vi "Test TDS1002 Oscilloscope API.vi"() -> ()   [LabVIEW 2020]
doc: "TDS1002 Oscilloscope API Tester."
uses:
  Support/Channel configuration--cluster.ctl
  Trigger config--cluster.ctl
  <vilib>/Utility/error.llb/DialogType.ctl
  TDS1002 Oscilloscope.lvlib
panel:
  in  "Timebase":dbl=0.0005
  in  "Configure timebase":bool
  out "Measurements":dbl(graph)
  in  "Measurement Type":i32(ring) items=["Frequency", "Mean", "Period", "Pulse Duty", "Peak to Peak", "Cycle RMS", "Minimum", "Maximum", "Rise Time", "Fall Time", "Positive Width", "Negative Width", "Amplitude", "Cycle Mean", "High", "Low", "Negative Duty", "Positive Overshoot", "Negative Overshoot", "Cursor Mean", "Burst Width", "Positive Pulse Count", "Negative Pulse Count", "Rising Edge Count", "Falling Edge Count", "Area", "Cycle Area", "RMS", "Cursor RMS"]
  in  "Channel":i32(ring)=1 items=["Channel 1"=1, "Channel 2"=2, "Channel 3"=3, "Channel 4"=4]
  in  "Get measurement":bool
  out "Data from display":waveform(dbl)(graph)
  in  "Stop continuous acquisition":bool
  in  "Timeout":i32
  in  "Start continuous acquistion":bool
  in  "Send software trigger":bool
  in  "Trigger config":T1 {"Trigger Coupling" items=["AC", "DC", "HF Reject", "LF Reject", "Noise Reject"]; "Trigger Slope" items=["Rising", "Falling"]; "Trigger Mode" items=["Auto", "Normal"]; "Trigger Source" items=["Channel 1", "Channel 2", "Channel 3", "Channel 4", "External Input", "Attenuated External Input"]}
  in  "Configure trigger":bool
  in  "Config parameters":T2={"Acquisition Type"=0, "Averaged Waveforms"=4, "Channel"=0, "Probe Attenuation"=10, "Timebase"=0.0005} {"Probe Attenuation" items=["1"=1, "10"=10, "20"=20, "50"=50, "100"=100, "500"=500, "1000"=1000]; "Channel" items=["Channel 1", "Channel 2", "Channel 3", "Channel 4", "Math", "Reference A", "Reference B", "Reference C", "Reference D"]; "Averaged Waveforms" items=["4"=4, "16"=16, "64"=64, "128"=128]; "Acquisition Type" items=["Sample", "Average", "Peak Detect"]}
  in  "Type":enum16{"On demand", "Continous"}(ring)
  in  "Configure":bool
  in  "Disconnect":bool
  in  "VISA resource name":refnum<visa-resource-name>
  in  "Connect":bool
  in  "Remove Panel from Subpanel":bool
  in  "Draw Panel into Subpanel":bool
  in  "Show Diagram on Init":bool
  in  "Run as Singleton?":bool
  in  "Show Block Diagram":bool
  in  "Refresh Modules":bool
  out "Active Modules":string[](array[string])
  in  "Stop Module":bool
  in  "Select Module":i32(ring)=-1 caption="Select Module\nTo send Request to" items=["All"=-1]
  in  "Run New Module":bool
  in  "Hide Module Panel":bool
  in  "Show Module Panel":bool
  out "Status":string
  # "This VI tests the API for the Module."
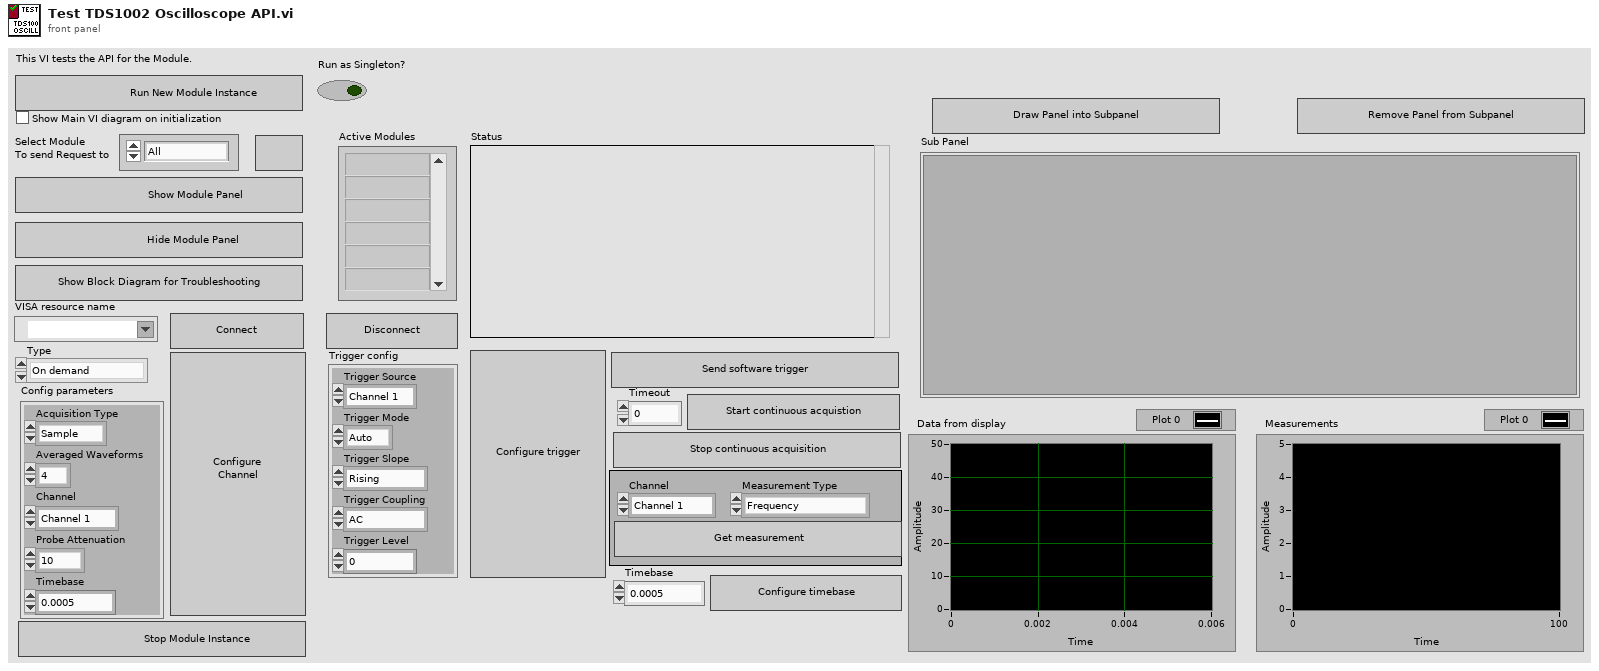
[diagram p1: front panel]
types:
  T1 = typedef "TDS1002 Oscilloscope.lvlib/Trigger config--cluster.ctl" = cluster{"Trigger Source":i32, "Trigger Mode":i32, "Trigger Slope":i32, "Trigger Coupling":i32, "Trigger Level":dbl}
  T2 = typedef "TDS1002 Oscilloscope.lvlib/Channel configuration--cluster.ctl" = cluster{"Acquisition Type":i32, "Averaged Waveforms":i32, "Channel":i32, "Probe Attenuation":i32, "Timebase":dbl}
  T3 = typedef "TDS1002 Oscilloscope.lvlib/Broadcast Events--cluster.ctl" = cluster{"Module Did Init":refnum<user-event>, "Status Updated":refnum<user-event>, "Error Reported":refnum<user-event>, "Module Did Stop":refnum<user-event>, "Update Module Execution Status":refnum<user-event>, "Helper Loop Status Updated":refnum<user-event>, "Device connected":refnum<user-event>, "Device disconnected":refnum<user-event>, "Data acquired":refnum<user-event>, "Configuration applied":refnum<user-event>}
  T4 = typedef "DialogType.ctl" = u16
  T5 = typedef "TDS1002 Oscilloscope.lvlib/Helper Loop Status--enum.ctl" = enum16{"Awake", "Asleep"}
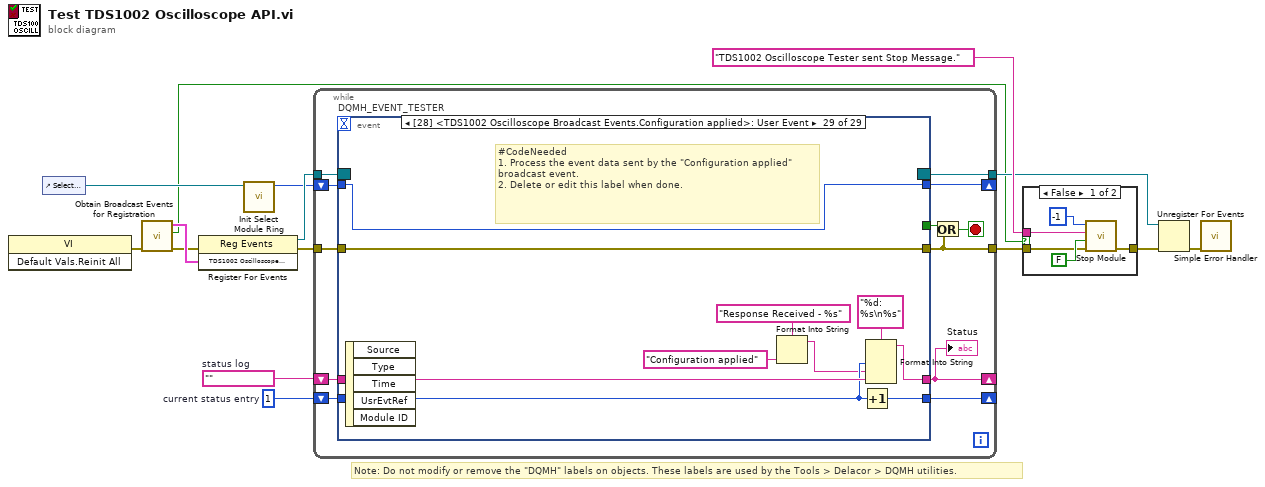
[diagram p0: block diagram]
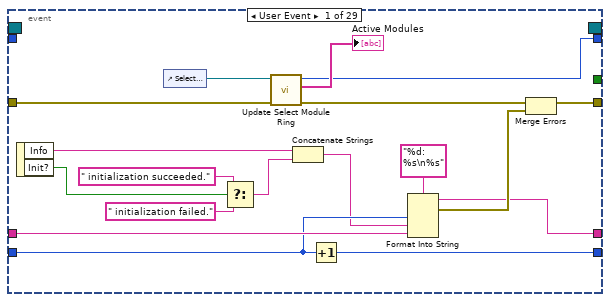
[diagram p3: hidden frame]
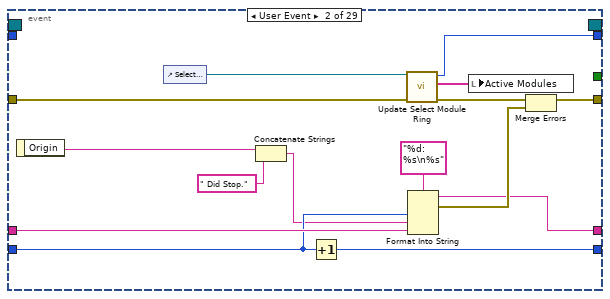
[diagram p4: hidden frame]
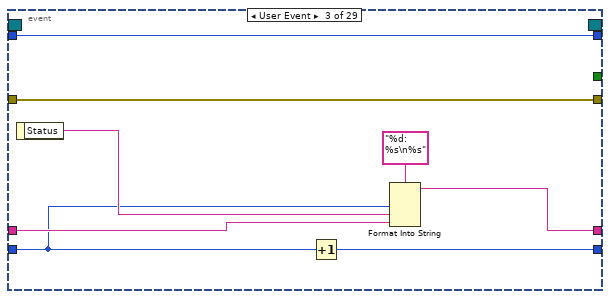
[diagram p5: hidden frame]
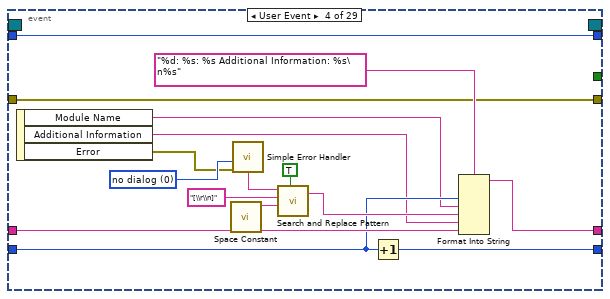
[diagram p6: hidden frame]
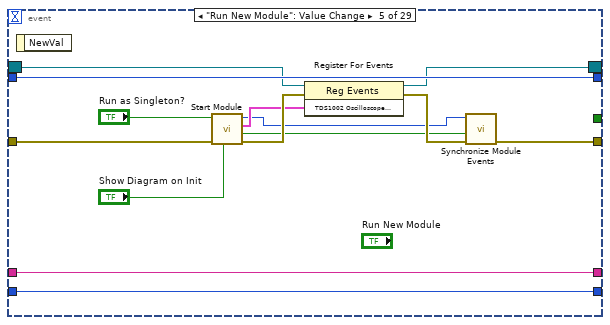
[diagram p7: hidden frame]
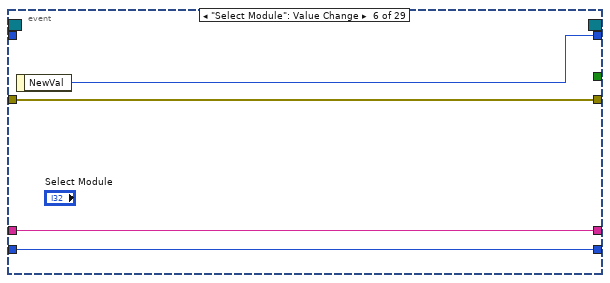
[diagram p8: hidden frame]
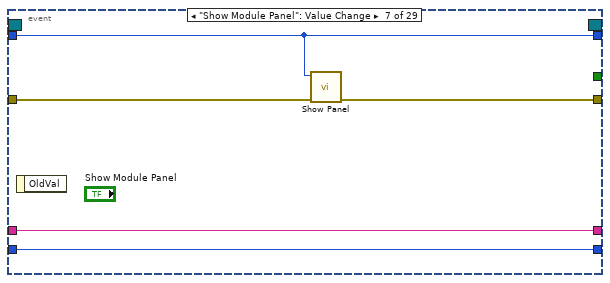
[diagram p9: hidden frame]
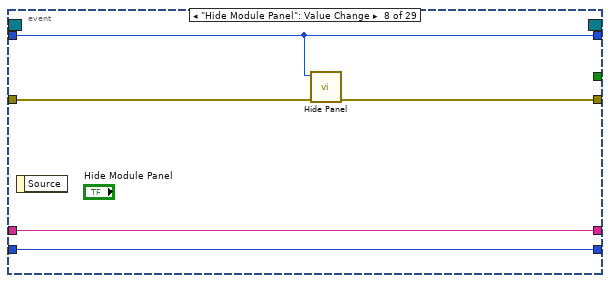
[diagram p10: hidden frame]
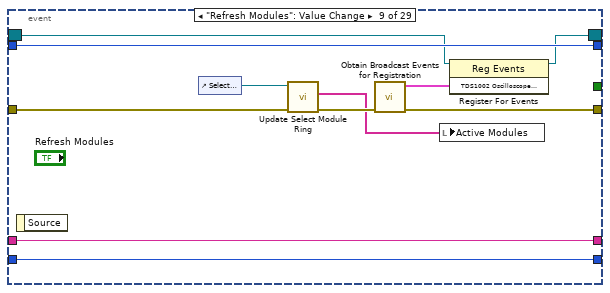
[diagram p11: hidden frame]
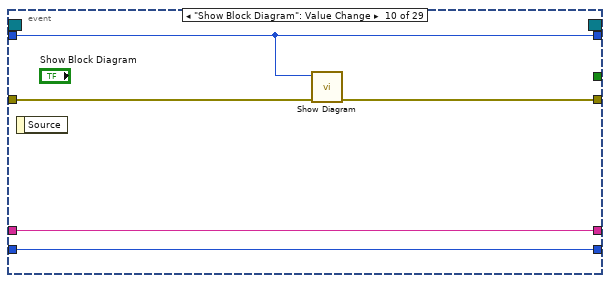
[diagram p12: hidden frame]
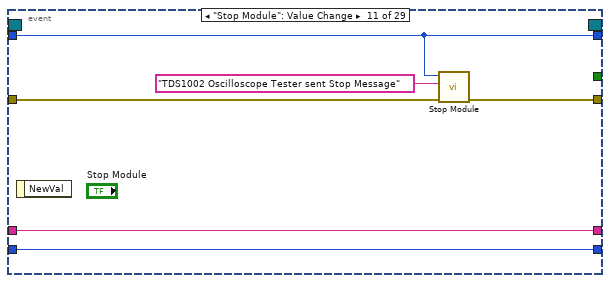
[diagram p13: hidden frame]
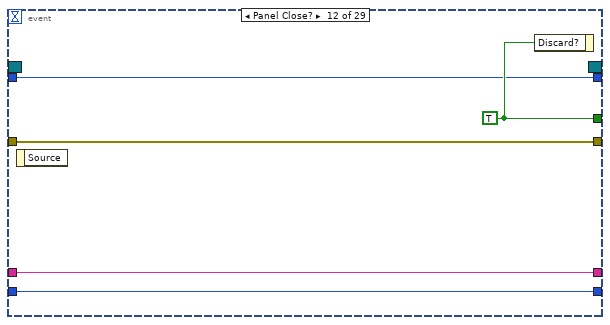
[diagram p14: hidden frame]
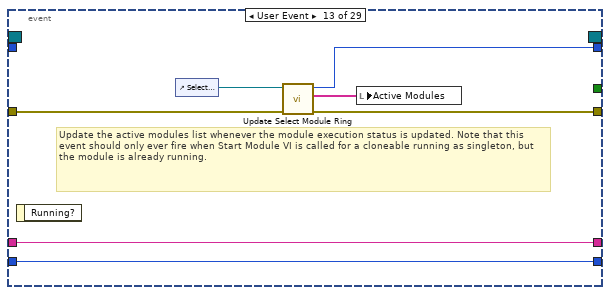
[diagram p15: hidden frame]
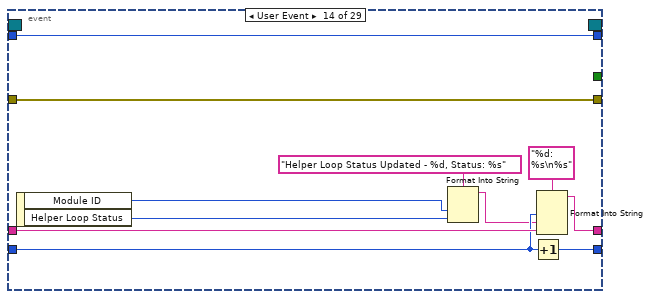
[diagram p16: hidden frame]
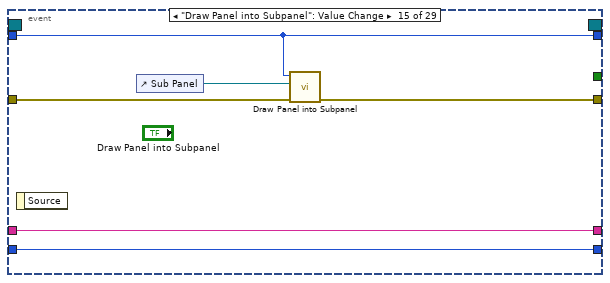
[diagram p17: hidden frame]
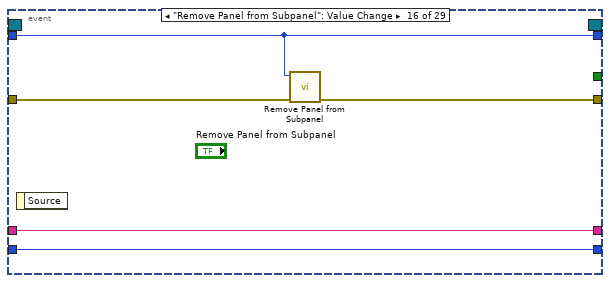
[diagram p18: hidden frame]
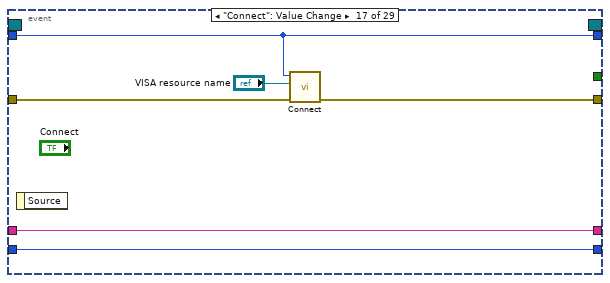
[diagram p19: hidden frame]
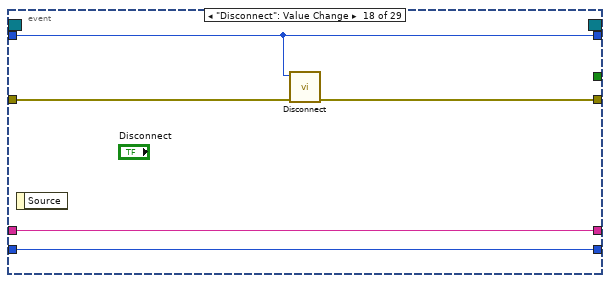
[diagram p20: hidden frame]
diagram:
  w12 = 1  # current status entry
  w13 = ""  # status log
  # "Note: Do not modify or remove the \"DQMH\" labels on objects. These labels are used by the Tools > Delacor > DQMH utilities."
  n1 = invoke class="VI" method="Default Vals.Reinit All"() -> (error out=w5:errorcluster)  [unwired: 3 in, 2 out]
  n2 = control-ref of="Select Module"() -> (w10:refnum<vi>)
  n3 = call "Obtain Broadcast Events for Registration.vi"("error in"=w5) -> ("error out"=w4:errorcluster, "Already running?"=w3:bool, "TDS1002 Oscilloscope Broadcast Events"=w9:T3)  [unwired: 8 in]
  n4 = register-events(error in=w4, w9) -> (reference out=w15:refnum<event-registration>, error out=w8:errorcluster)  [unwired: 1 in]
  n5 = call "Init Select Module Ring.vi"("Select Module Ring Ref"=w10) -> ("Value for All Modules"=w11:i32)  [unwired: 8 in, 2 out]
  n6 = while {
    tunnel: w15 -> [w27]
    tunnel: [w16] -> w2
    tunnel: w8 -> [w25]
    shift-right: [w21] -> _
    shift-left: w13 -> [w23]
    shift-right: [w22] -> _
    shift-left: w12 -> [w24]
    shift-right: [w18] -> _
    shift-left: w11 -> [w19]
    tunnel: [w17] -> w6
    stop <- w20 stop-if-true
    n7 = event "DQMH_EVENT_TESTER" shown="[28] <TDS1002 Oscilloscope Broadcast Events.Configuration applied>: User Event" {
      selector: w27 -> [_ _ _ _ w92 _ _ _ w118 _ _ _ _ _ _ _ _ _ _ _ _ _ _ _ _ _ _ _ _]
      dyn-events: [_ _ _ _ w91 _ _ _ w117 _ _ _ _ _ _ _ _ _ _ _ _ _ _ _ _ _ _ _ _] -> w17
      timeout: _ -> [_ _ _ _ _ _ _ _ _ _ _ _ _ _ _ _ _ _ _ _ _ _ _ _ _ _ _ _ _]
      tunnel: [_ _ _ _ _ _ _ _ _ _ _ w139 _ _ _ _ _ _ _ _ _ _ _ _ _ _ _ _ _] -> w26
      tunnel: [w35 w52 w68 w72 w90 w102 w106 w111 w114 w125 w130 w138 w142 w157 w160 w165 w171 w176 w189 w199 w203 w209 w214 w228 w231 w236 w244 w250 w263] -> w16
      tunnel: w25 -> [w37 w54 w68 w72 w93 w102 w107 w112 w119 w128 w131 w138 w143 w157 w163 w168 w174 w179 w189 w199 w206 w212 w217 w228 w234 w239 w247 w253 w263]
      tunnel: w24 -> [w42 w57 w61 w75 w95 w100 w104 w109 w122 w126 w133 w136 w145 w153 w161 w166 w172 w177 w185 w195 w204 w210 w215 w224 w232 w237 w245 w251 w259]
      tunnel: w23 -> [w43 w58 w64 w76 w96 w101 w105 w110 w123 w127 w134 w137 w146 w155 w162 w167 w173 w178 w187 w197 w205 w211 w216 w226 w233 w238 w246 w252 w261]
      tunnel: [w40 w55 w65 w74 w96 w101 w105 w110 w123 w127 w134 w137 w146 w154 w162 w167 w173 w178 w186 w196 w205 w211 w216 w225 w233 w238 w246 w252 w260] -> w21
      tunnel: [w41 w56 w67 w73 w95 w100 w104 w109 w122 w126 w133 w136 w145 w152 w161 w166 w172 w177 w184 w194 w204 w210 w215 w223 w232 w237 w245 w251 w258] -> w22
      tunnel: w19 -> [_ _ w62 w84 w94 _ w103 w108 w121 w124 w132 w135 _ w156 w159 w164 w170 w175 w188 w198 w202 w208 w213 w227 w230 w235 w243 w249 w262]
      tunnel: [w32 w49 w62 w84 w94 w99 w103 w108 w121 w124 w132 w135 w141 w156 w159 w164 w170 w175 w188 w198 w202 w208 w213 w227 w230 w235 w243 w249 w262] -> w18
      event User Event {
        n8 = event-data() -> ("Info"=w39:string, "Init?"=w29:bool)  [unwired: 1 in]
        n9 = control-ref of="Select Module"() -> (w34:refnum<vi>)
        n10 = Select(t=" initialization succeeded.", s=w29, f=" initialization failed.") -> (s? t:f=w28:string)
        n11 = call "Update Select Module Ring.vi"("error in (no error)"=w37, "Select Module Ring Ref"=w34) -> ("error out"=w36:errorcluster, "Active Modules (Array)"=→"Active Modules":string[], "New Module Ring Value"=w32:i32)  [unwired: 7 in]
        n12 = Concatenate Strings(w39, w28) -> (w38:string)
        n13 = Increment(x=w42) -> (x+1=w41:i32)
        n14 = Format Into String(format string="%d: %s\n%s", w42, w38, w43) -> (resulting string=w40:string, error out=w45:errorcluster)  [unwired: 2 in]
        n15 = Merge Errors(w36, w45) -> (w35:errorcluster)
      }
      event User Event {
        n16 = event-data() -> ("Origin"=w47:string)  [unwired: 1 in]
        n17 = control-ref of="Select Module"() -> (w51:refnum<vi>)
        n18 = Concatenate Strings(w47, " Did Stop.") -> (w46:string)
        n19 = Increment(x=w57) -> (x+1=w56:i32)
        n20 = call "Update Select Module Ring.vi"("error in (no error)"=w54, "Select Module Ring Ref"=w51) -> ("error out"=w53:errorcluster, "Active Modules (Array)"=w50:string[], "New Module Ring Value"=w49:i32)  [unwired: 7 in]
        n21 = Format Into String(format string="%d: %s\n%s", w57, w46, w58) -> (resulting string=w55:string, error out=w60:errorcluster)  [unwired: 2 in]
        n22 = local write "Active Modules"(w50) -> ()
        n23 = Merge Errors(w53, w60) -> (w52:errorcluster)
      }
      event User Event {
        n24 = event-data() -> ("Status"=w63:string)  [unwired: 1 in]
        n25 = Increment(x=w61) -> (x+1=w67:i32)
        n26 = Format Into String(format string="%d: %s\n%s", w61, w63, w64) -> (resulting string=w65:string)  [unwired: 2 in, 1 out]
      }
      event User Event {
        w77 = T4 0 items=["no dialog", "OK message", "continue or stop message", "OK message + warnings", "continue/stop + warnings"] ("type of dialog (OK msg:1)")
        n27 = event-data() -> ("Module Name"=w71:string, "Additional Information"=w70:string, "Error"=w69:errorcluster)  [unwired: 1 in]
        n28 = call <vilib>:"Space Constant.vi"() -> ("String"=w81:string)
        n29 = call <vilib>:"Simple Error Handler.vi"("type of dialog (OK msg:1)"=w77, "error in (no error)"=w69) -> ("message"=w78:string)  [unwired: 3 in, 4 out]
        n30 = call <vilib>:"Search and Replace Pattern.vi"("string"=w78, "regular expression (\"\")"="[\\r\\n]" ("regular expression (\"\")"), "replace string (\"\")"=w81, "replace all? (F)"=TRUE ("replace all CR/LF with spaces")) -> ("result string"=w79:string)  [unwired: 1 in, 1 out]
        n31 = Increment(x=w75) -> (x+1=w73:i32)
        n32 = Format Into String(format string="%d: %s: %s Additional Information: %s\n%s", w75, w71, w79, w70, w76) -> (resulting string=w74:string)  [unwired: 2 in, 1 out]
      }
      event "Run New Module": Value Change {
        n33 = event-data() -> ()  [unwired: 1 in, 1 out]
        n34 = call "Start Module.vi"("Show Main VI Diagram on Init (F)"="Show Diagram on Init", "error in"=w93, "Run as Singleton? (F)"="Run as Singleton?") -> ("error out"=w97:errorcluster, "Wait for Event Sync?"=w89:bool, "TDS1002 Oscilloscope Broadcast Events"=w88:T3, "Module ID"=w85:i32)  [unwired: 5 in]
        n35 = register-events(reference=w92, error in=w97, w88) -> (reference out=w91:refnum<event-registration>, error out=w98:errorcluster)
        n36 = call "Synchronize Module Events.vi"("error in"=w98, "Wait for Event Sync?"=w89, "Module ID in"=w85) -> ("error out"=w90:errorcluster)  [unwired: 7 in, 1 out]
      }
      event "Select Module": Value Change {
        n37 = event-data() -> ("NewVal"=w99:i32)  [unwired: 1 in]
      }
      event "Show Module Panel": Value Change {
        n38 = event-data() -> ()  [unwired: 1 in, 1 out]
        n39 = call "Show Panel.vi"("error in (no error)"=w107, "Module ID"=w103) -> ("error out"=w106:errorcluster)  [unwired: 9 in]
      }
      event "Hide Module Panel": Value Change {
        n40 = event-data() -> ()  [unwired: 1 in, 1 out]
        n41 = call "Hide Panel.vi"("error in (no error)"=w112, "Module ID"=w108) -> ("error out"=w111:errorcluster)  [unwired: 9 in]
      }
      event "Refresh Modules": Value Change {
        n42 = event-data() -> ()  [unwired: 1 in, 1 out]
        n43 = control-ref of="Select Module"() -> (w120:refnum<vi>)
        n44 = call "Update Select Module Ring.vi"("error in (no error)"=w119, "Select Module Ring Ref"=w120) -> ("error out"=w115:errorcluster, "Active Modules (Array)"=w113:string[])  [unwired: 7 in, 1 out]
        n45 = call "Obtain Broadcast Events for Registration.vi"("error in"=w115) -> ("error out"=w114:errorcluster, "TDS1002 Oscilloscope Broadcast Events"=w116:T3)  [unwired: 8 in, 1 out]
        n46 = local write "Active Modules"(w113) -> ()
        n47 = register-events(reference=w118, w116) -> (reference out=w117:refnum<event-registration>)  [unwired: 1 in, 1 out]
      }
      event "Show Block Diagram": Value Change {
        n48 = event-data() -> ()  [unwired: 1 in, 1 out]
        n49 = call "Show Diagram.vi"("error in (no error)"=w128, "Module ID"=w124) -> ("error out"=w125:errorcluster)  [unwired: 9 in]
      }
      event "Stop Module": Value Change {
        n50 = event-data() -> ()  [unwired: 1 in, 1 out]
        n51 = call "Stop Module.vi"("error in"=w131, "Origin"="TDS1002 Oscilloscope Tester sent Stop Message", "Module ID"=w132) -> ("error out"=w130:errorcluster)  [unwired: 8 in]
      }
      event Panel Close? {
        w139 = TRUE ("Discard?")
        n52 = event-data() -> ()  [unwired: 1 in, 1 out]
        n53 = event-data("Discard?"=w139) -> ()  [unwired: 1 in, 1 out]
      }
      event User Event {
        # "Update the active modules list whenever the module execution status is updated. Note that this event should only ever fire when Start Module VI is called for a cloneable running as singleton, but the module is already running."
        n54 = event-data() -> ()  [unwired: 1 in, 1 out]
        n55 = control-ref of="Select Module"() -> (w144:refnum<vi>)
        n56 = call "Update Select Module Ring.vi"("error in (no error)"=w143, "Select Module Ring Ref"=w144) -> ("error out"=w142:errorcluster, "Active Modules (Array)"=w140:string[], "New Module Ring Value"=w141:i32)  [unwired: 7 in]
        n57 = local write "Active Modules"(w140) -> ()
      }
      event User Event {
        n58 = event-data() -> ("Module ID"=w148:i32, "Helper Loop Status"=w147:T5)  [unwired: 1 in]
        n59 = Format Into String(format string="Helper Loop Status Updated - %d, Status: %s", w148, w147) -> (resulting string=w149:string)  [unwired: 2 in, 1 out]
        n60 = Increment(x=w153) -> (x+1=w152:i32)
        n61 = Format Into String(format string="%d: %s\n%s", w153, w149, w155) -> (resulting string=w154:string)  [unwired: 2 in, 1 out]
      }
      event "Draw Panel into Subpanel": Value Change {
        n62 = event-data() -> ()  [unwired: 1 in, 1 out]
        n63 = control-ref of="Sub Panel"() -> (w158:refnum<vi>)
        n64 = call "Draw Panel into Subpanel.vi"("error in"=w163, "Sub Panel"=w158, "Module ID"=w159) -> ("error out"=w160:errorcluster)  [unwired: 8 in]
      }
      event "Remove Panel from Subpanel": Value Change {
        n65 = event-data() -> ()  [unwired: 1 in, 1 out]
        n66 = call "Remove Panel from Subpanel.vi"("error in"=w168, "Module ID"=w164) -> ("error out"=w165:errorcluster)  [unwired: 9 in]
      }
      event "Connect": Value Change {
        n67 = event-data() -> ()  [unwired: 1 in, 1 out]
        n68 = call "Connect.vi"("error in"=w174, "VISA resource name"="VISA resource name", "Module ID"=w170) -> ("error out"=w171:errorcluster)  [unwired: 8 in]
      }
      event "Disconnect": Value Change {
        n69 = event-data() -> ()  [unwired: 1 in, 1 out]
        n70 = call "Disconnect.vi"("error in"=w179, "Module ID"=w175) -> ("error out"=w176:errorcluster)  [unwired: 9 in]
      }
      event User Event {
        n71 = event-data() -> ()  [unwired: 1 in, 5 out]
        n72 = Format Into String(format string="Response Received - %s", "Connection to device successful." ("input 1")) -> (resulting string=w181:string)  [unwired: 2 in, 1 out]
        n73 = Increment(x=w185) -> (x+1=w184:i32)
        n74 = Format Into String(format string="%d: %s\n%s", w185, w181, w187) -> (resulting string=w186:string)  [unwired: 2 in, 1 out]
      }
      event User Event {
        n75 = event-data() -> ()  [unwired: 1 in, 5 out]
        n76 = Format Into String(format string="Response Received - %s", "Device disconnected." ("input 1")) -> (resulting string=w191:string)  [unwired: 2 in, 1 out]
        n77 = Increment(x=w195) -> (x+1=w194:i32)
        n78 = Format Into String(format string="%d: %s\n%s", w195, w191, w197) -> (resulting string=w196:string)  [unwired: 2 in, 1 out]
      }
      event "Configure": Value Change {
        n79 = event-data() -> ()  [unwired: 1 in, 1 out]
        n80 = call "Configure acquisition.vi"("Config parameters"="Config parameters", "error in"=w206, "Type"="Type", "Module ID"=w202) -> ("error out"=w203:errorcluster)  [unwired: 7 in]
      }
      event "Configure trigger": Value Change {
        n81 = event-data() -> ()  [unwired: 1 in, 1 out]
        n82 = call "Configure trigger.vi"("error in"=w212, "Trigger config"="Trigger config", "Module ID"=w208) -> ("error out"=w209:errorcluster)  [unwired: 8 in]
      }
      event "Send software trigger": Value Change {
        n83 = event-data() -> ()  [unwired: 1 in, 1 out]
        n84 = call "Send software trigger.vi"("error in"=w217, "Module ID"=w213) -> ("error out"=w214:errorcluster)  [unwired: 9 in]
      }
      event User Event {
        n85 = event-data() -> ("Waveform"=→"Data from display":waveform(dbl))  [unwired: 1 in, 4 out]
        n86 = Format Into String(format string="Response Received - %s", "Data acquired" ("input 1")) -> (resulting string=w220:string)  [unwired: 2 in, 1 out]
        n87 = Increment(x=w224) -> (x+1=w223:i32)
        n88 = Format Into String(format string="%d: %s\n%s", w224, w220, w226) -> (resulting string=w225:string)  [unwired: 2 in, 1 out]
      }
      event "Start continuous acquistion": Value Change {
        n89 = event-data() -> ()  [unwired: 1 in, 1 out]
        n90 = call "Start continuous acquistion.vi"("error in"=w234, "Timeout"="Timeout", "Module ID"=w230) -> ("error out"=w231:errorcluster)  [unwired: 8 in]
      }
      event "Stop continuous acquisition": Value Change {
        n91 = event-data() -> ()  [unwired: 1 in, 1 out]
        n92 = call "Stop continuous acquisition.vi"("error in"=w239, "Module ID"=w235) -> ("error out"=w236:errorcluster)  [unwired: 9 in]
      }
      event "Get measurement": Value Change {
        n93 = event-data() -> ()  [unwired: 1 in, 1 out]
        n94 = call "Get measurement.vi"("error in"=w247, "Measurement Type"="Measurement Type", "Channel"="Channel", "Module ID"=w243) -> ("error out"=w244:errorcluster, "Value"=→"Measurements":dbl)  [unwired: 5 in, 1 out]
      }
      event "Configure timebase": Value Change {
        n95 = event-data() -> ()  [unwired: 1 in, 1 out]
        n96 = call "Configure timebase.vi"("error in"=w253, "Timebase"="Timebase", "Module ID"=w249) -> ("error out"=w250:errorcluster)  [unwired: 8 in]
      }
      event User Event {
        # "#CodeNeeded\n1. Process the event data sent by the \"Configuration applied\" broadcast event.\n2. Delete or edit this label when done."
        n97 = event-data() -> ()  [unwired: 1 in, 5 out]
        n98 = Format Into String(format string="Response Received - %s", "Configuration applied" ("input 1")) -> (resulting string=w255:string)  [unwired: 2 in, 1 out]
        n99 = Increment(x=w259) -> (x+1=w258:i32)
        n100 = Format Into String(format string="%d: %s\n%s", w259, w255, w261) -> (resulting string=w260:string)  [unwired: 2 in, 1 out]
      }
    }
    "Status" <- w21
    n101 = Or(x=w26, y=w16) -> (x .or. y?=w20:bool)
  }
  n102 = case shown="False" w3 {
    tunnel: [w268 w269] -> w14
    tunnel: "TDS1002 Oscilloscope Tester sent Stop Message." ("Origin") -> [w267 _]
    tunnel: w2 -> [w264 w269]
    frame False {
      n103 = call "Stop Module.vi"("error in"=w264, "Wait for Module to stop? (F)"=FALSE ("Wait for Module to stop?"), "Origin"=w267, "Module ID"=-1 ("Stop all")) -> ("error out"=w268:errorcluster)  [unwired: 7 in]
    }
    frame True {
    }
  }
  n104 = Unregister For Events(event registration refnum=w6, error in=w14) -> (error out=w1:errorcluster)
  n105 = call <vilib>:"Simple Error Handler.vi"("error in (no error)"=w1) -> ()  [unwired: 4 in, 5 out]
